vi "Unit Test.vi"() -> ()   [LabVIEW 2018]
uses:
  NRT8000.lvclass
  PPLs/Optical Spectrum Analyzer/Parent/OSA.lvlibp/Optical Spectrum Analyzer.lvclass
  C:/Projects/LabVIEW/PPLs/Optical Spectrum Analyzer/Parent/OSA.lvlibp/Optical Spectrum Analyzer.lvclass
panel:
  out "error out 2":errorcluster
  in  "Cmd":string="*IDN?"
  out "Rsp":string
  in  "Command":bool
  out "Manufacturer Name":string
  out "Device Name":string
  out "Serial Number":string
  out "Firmware Revision":string
  out "error out":errorcluster
  in  "stop":bool
  in  "Get ID":bool
  in  "error in (no error)":errorcluster
  in  "Resource":refnum<visa-resource-name>
  # "1"
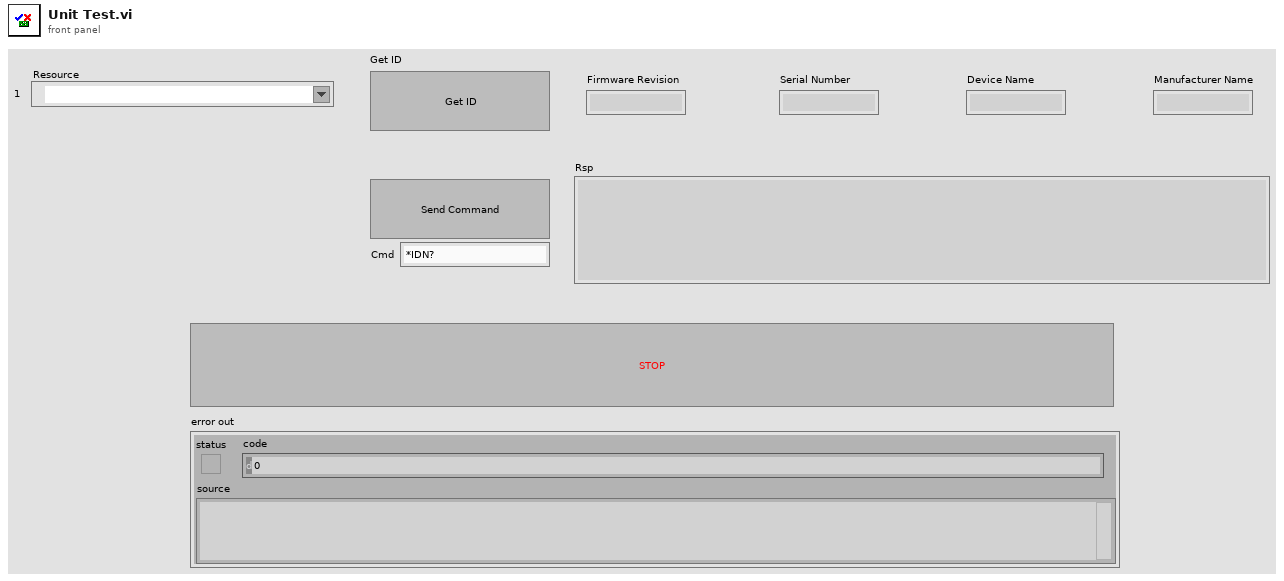
[diagram p1: front panel]
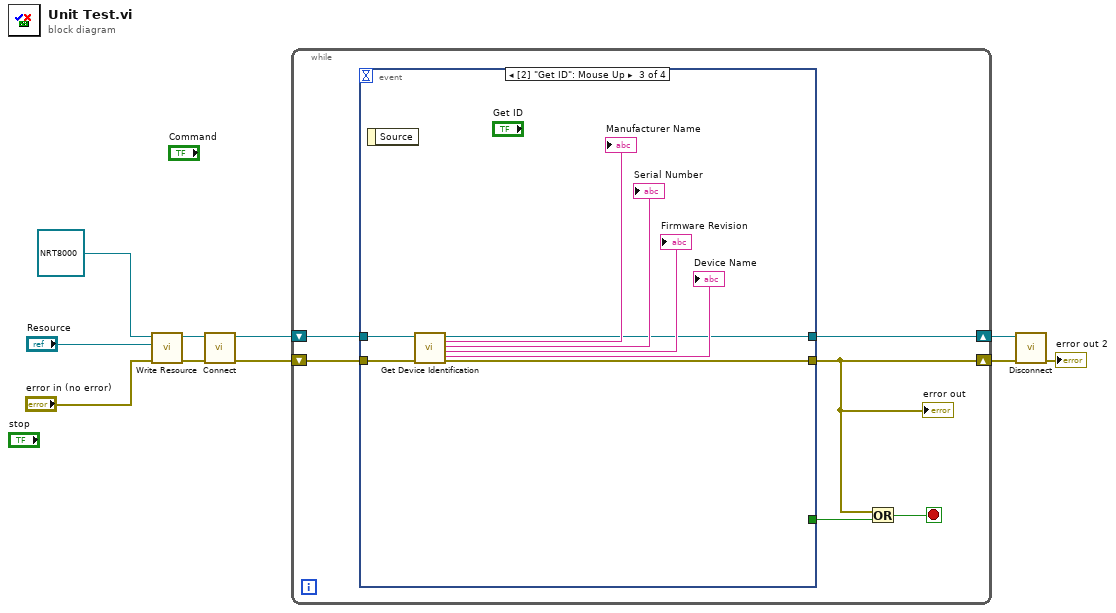
[diagram p0: block diagram]
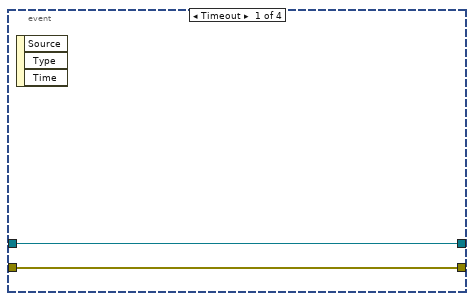
[diagram p2: hidden frame]
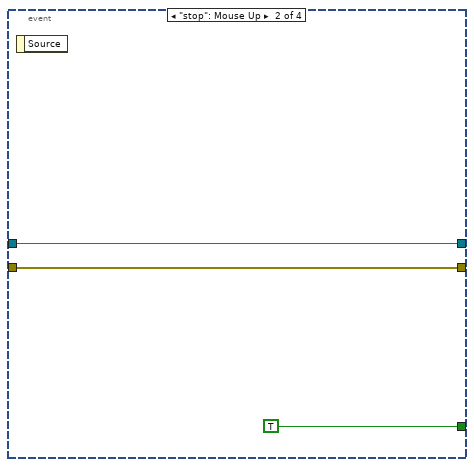
[diagram p3: hidden frame]
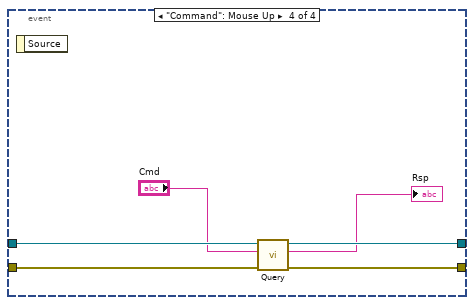
[diagram p4: hidden frame]
diagram:
  n1 = call "Write Resource.vi"("error in (no error)"="error in (no error)", "Resource"="Resource", "Optical Spectrum Analyzer in"=refnum<class "NRT8000.lvclass"> refnum ("NRT8000.lvlib:NRT8000.lvclass")) -> ("error out"=w6:errorcluster, "Optical Spectrum Analyzer out"=w7:refnum<class "NRT8000.lvclass">)  [unwired: 7 in]
  n2 = call-dynamic "Connect.vi"("error in (no error)"=w6, "NRT8000 in"=w7) -> ("error out"=w4:errorcluster, "NRT8000 out"=w5:refnum<class "NRT8000.lvclass">)  [unwired: 8 in]
  n3 = while {
    shift-right: [w14] -> w3
    shift-left: w5 -> [w16]
    shift-right: [w13] -> w2
    shift-left: w4 -> [w15]
    stop <- w11 stop-if-true
    n4 = event shown="[2] \"Get ID\": Mouse Up" {
      selector: _ -> [_ _ _ _]
      dyn-events: _ -> [_ _ _ _]
      timeout: _ -> [_ _ _ _]
      tunnel: w16 -> [w18 w20 w29 w35]
      tunnel: w15 -> [w17 w19 w28 w34]
      tunnel: [_ TRUE _ _] -> w12
      tunnel: [w18 w20 w22 w33] -> w14
      tunnel: [w17 w19 w23 w30] -> w13
      event Timeout {
        n5 = event-data() -> ()  [unwired: 1 in, 3 out]
      }
      event "stop": Mouse Up {
        n6 = event-data() -> ()  [unwired: 1 in, 1 out]
      }
      event "Get ID": Mouse Up {
        n7 = event-data() -> ()  [unwired: 1 in, 1 out]
        n8 = call-dynamic "Get Device Identification.vi"("error in (no error)"=w28, "NRT8000 in"=w29) -> ("error out"=w23:errorcluster, "Firmware Revision"=→"Firmware Revision":string, "Serial Number"=→"Serial Number":string, "NRT8000 out"=w22:refnum<class "NRT8000.lvclass">, "Device Name"=→"Device Name":string, "Manufacturer Name"=→"Manufacturer Name":string)  [unwired: 4 in]
      }
      event "Command": Mouse Up {
        n9 = event-data() -> ()  [unwired: 1 in, 1 out]
        n10 = call "Query.vi"("error in (no error)"=w34, "Cmd"="Cmd", "NRT8000 in"=w35) -> ("error out"=w30:errorcluster, "Rsp"=→"Rsp":string, "NRT8000 out"=w33:refnum<class "NRT8000.lvclass">)  [unwired: 6 in]
      }
    }
    "error out" <- w13
    n11 = Or(x=w13, y=w12) -> (x .or. y?=w11:bool)
  }
  n12 = call-dynamic "Disconnect.vi"("error in (no error)"=w2, "NRT8000 in"=w3) -> ("error out"=→"error out 2":errorcluster)  [unwired: 8 in, 1 out]
